vi "test boucle For.vi"() -> ()   [LabVIEW 2024]
panel:
  out "Tableau 2":i32[](array[numeric])
  out "x/y":dbl
  out "x+y":i32
  out "Tableau":i32[](array[numeric])
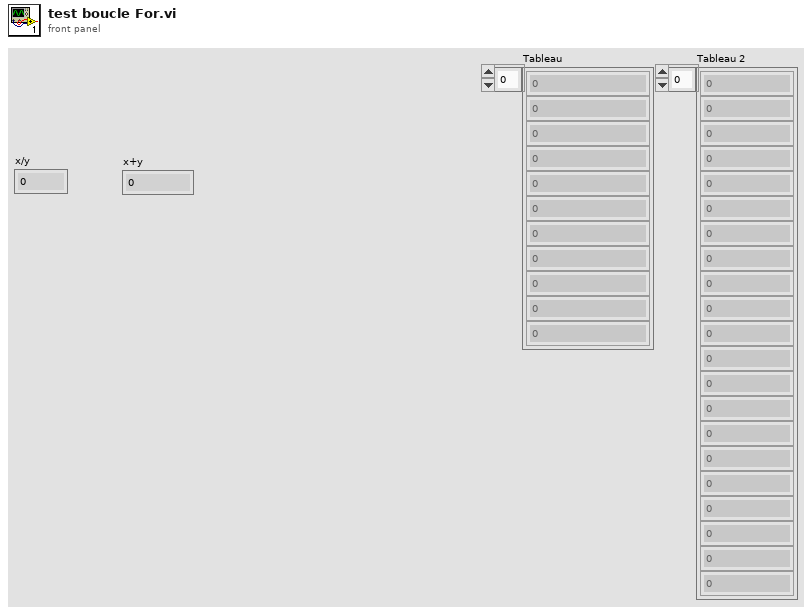
[diagram p1: front panel]
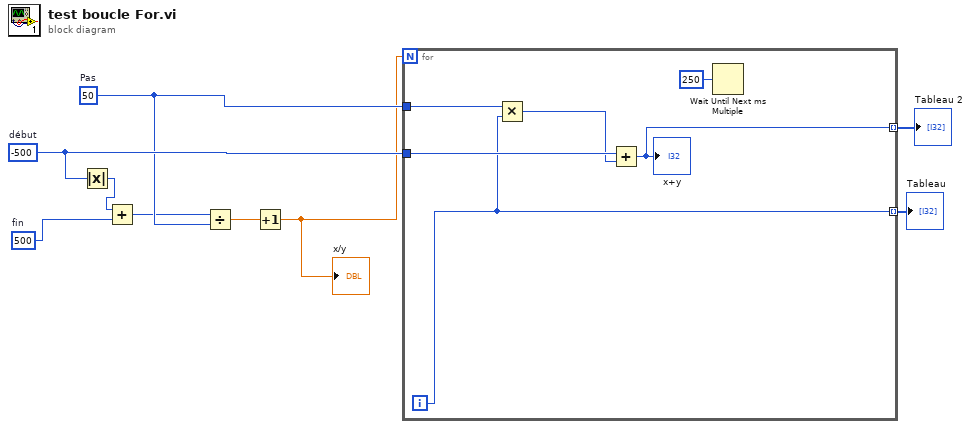
[diagram p0: block diagram]
diagram:
  w6 = 500  # fin
  w5 = 50  # Pas
  w8 = -500  # début
  n1 = Absolute Value(x=w8) -> (abs(x)=w7:i32)
  n2 = Add(x=w7, y=w6) -> (x+y=w4:i32)
  n3 = Divide(x=w4, y=w5) -> (x/y=w3:dbl)
  n4 = Increment(x=w3) -> (x+1=w1:dbl)
  "x/y" <- w1
  n5 = for {
    N: w1 -> [_]
    tunnel: [w14] -> w9 mode=indexing
    tunnel: w8 -> [w15]
    tunnel: w5 -> [w13]
    tunnel: [w10] -> w2 mode=indexing
    i -> [w14]
    n6 = Multiply(x=w13, y=w14) -> (x*y=w12:i32)
    n7 = Add(x=w15, y=w12) -> (x+y=w10:i32)
    "x+y" <- w10
    n8 = Wait Until Next ms Multiple(millisecond multiple=u32 250 ("n millisecondes")) -> ()  [unwired: 1 out]
  }
  "Tableau" <- w9
  "Tableau 2" <- w2
